vi "Teleop.vi"(10 "Match Info":T1={"Autonomous Elapsed Seconds"=0.0, "TeleOp Elapsed Seconds"=0.0, "Disabled Elapsed Seconds"=0.0, "Visited Autonomous"=FALSE, "Visited TeleOp"=FALSE, "Visited Disabled"=FALSE, "Autonomous Settings"={"Autonomous Style"=enum."Independent", "VI Refnum"=refnum}}, 11 "Call Context":T2) -> ()   [LabVIEW 2017]
doc: "This VI is called for each TeleOp packet received from the DS where the robot is not disabled. It is often used to read from the joysticks and update I/O or to update setpoints for timed control loops. It should complete and return within 20 milliseconds or it may miss DS packets."
uses:
  <vilib>/Rock Robotics/WPI/DriverStation/WPI_DriverStationDerivedRobotMode.ctl
  <vilib>/Rock Robotics/WPI/DriverStation/WPI_DriverStationMatch Info.ctl
  <vilib>/Rock Robotics/WPI/Utilities/WPI_GetSetVariantRefNum.vi
  <vilib>/Rock Robotics/Network Tables/NT Write Boolean Array.vi
  <vilib>/Rock Robotics/Network Tables/NT Write Numeric Array.vi
  <vilib>/Rock Robotics/Network Tables/NT Read Boolean.vi
  <vilib>/Rock Robotics/Network Tables/NT Read Number.vi
panel:
  out "Sample Boolean 3":bool
  out "Sample Boolean 2":bool
  out "Sample Slider 1":dbl(slide) scale=0.0..5.0
  out "Left axis value":dbl
  out "Right axis value":dbl
  in  "Square Inputs":bool
  out "Left Motor Value":dbl
  out "Right Motor Value":dbl
  in  "Max Output":dbl
  out "Sample Slider 0":dbl(slide) scale=0.0..5.0
  out "Sample Boolean 1":bool
  out "Sample Boolean 0":bool
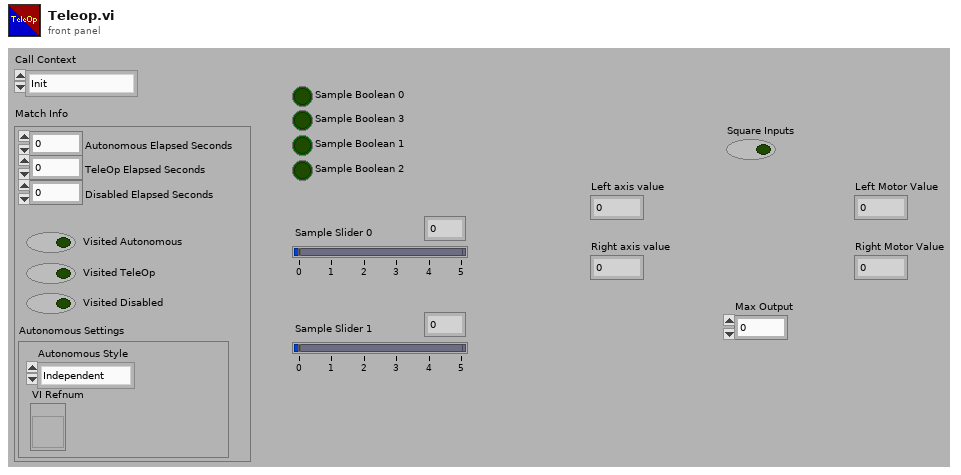
[diagram p1: front panel]
types:
  T1 = typedef "WPI_DriverStationMatch Info.ctl" = cluster{"Autonomous Elapsed Seconds":dbl, "TeleOp Elapsed Seconds":dbl, "Disabled Elapsed Seconds":dbl, "Visited Autonomous":bool, "Visited TeleOp":bool, "Visited Disabled":bool, "Autonomous Settings":cluster{"Autonomous Style":enum16{"Iterative", "Independent"}, "VI Refnum":refnum<vi>}}
  T2 = typedef "WPI_DriverStationDerivedRobotMode.ctl" = enum16{"Init", "Execute", "Stop"}
  T3 = typedef "WPI_JoystickDevRef.ctl" = cluster{"Device":T4}
  T4 = typedef "WPI_JoystickDeviceEnum.ctl" = enum16{"USB 0", "USB 1", "USB 2", "USB 3", "USB 4", "USB 5"}
  T5 = typedef "WPI_MotorControlDeviceRef.ctl" = cluster{"DeviceStatus":errorcluster, "Type":T6, "PWM":cluster{"PWM Channel":T7, "DeadBand":T8}, "CAN":cluster{"Device Number":u8, "SetOutput VI Ref":variant, "GetOutput VI Ref":variant, "Enable VI Ref":variant, "Disable VI Ref":variant, "Data":variant}, "Invert":bool, "DIO PWM":cluster{"PWM \"Enable\" Channel":T7, "DIOChannel":T9, "PWM Rate":dbl}}
  T6 = typedef "WPI_MotorControlType.ctl" = enum16{"PWM", "CAN", "DIO PWM"}
  T7 = typedef "FPGA_DIOPWMChannel.ctl" = enum8{"PWM 0", "PWM 1", "PWM 2", "PWM 3", "PWM 4", "PWM 5", "PWM 6", "PWM 7", "PWM 8", "PWM 9", "PWM MXP 0", "PWM MXP 1", "PWM MXP 2", "PWM MXP 3", "PWM MXP 4", "PWM MXP 5", "PWM MXP 6", "PWM MXP 7", "PWM MXP 8", "PWM MXP 9", "Invalid"}
  T8 = typedef "WPI_PWMDeadband.ctl" = cluster{"Name":string, "maxPositivePwm":i32, "minPositivePwm":i32, "centerPwm":i32, "maxNegativePwm":i32, "minNegativePwm":i32, "angularRange":u16}
  T9 = typedef "FPGA_DIOChannel.ctl" = enum8{"DIO 0", "DIO 1", "DIO 2", "DIO 3", "DIO 4", "DIO 5", "DIO 6", "DIO 7", "DIO 8", "DIO 9", "DIO MXP 0", "DIO MXP 1", "DIO MXP 2", "DIO MXP 3", "DIO MXP 4", "DIO MXP 5", "DIO MXP 6", "DIO MXP 7", "DIO MXP 8", "DIO MXP 9", "DIO MXP 10", "DIO MXP 11", "DIO MXP 12", "DIO MXP 13", "DIO MXP 14", "DIO MXP 15", "SPI Port CS1", "SPI Port CS2", "SPI Port CS3", "SPI Port MISO", "SPI Port MOSI", "Invalid"}
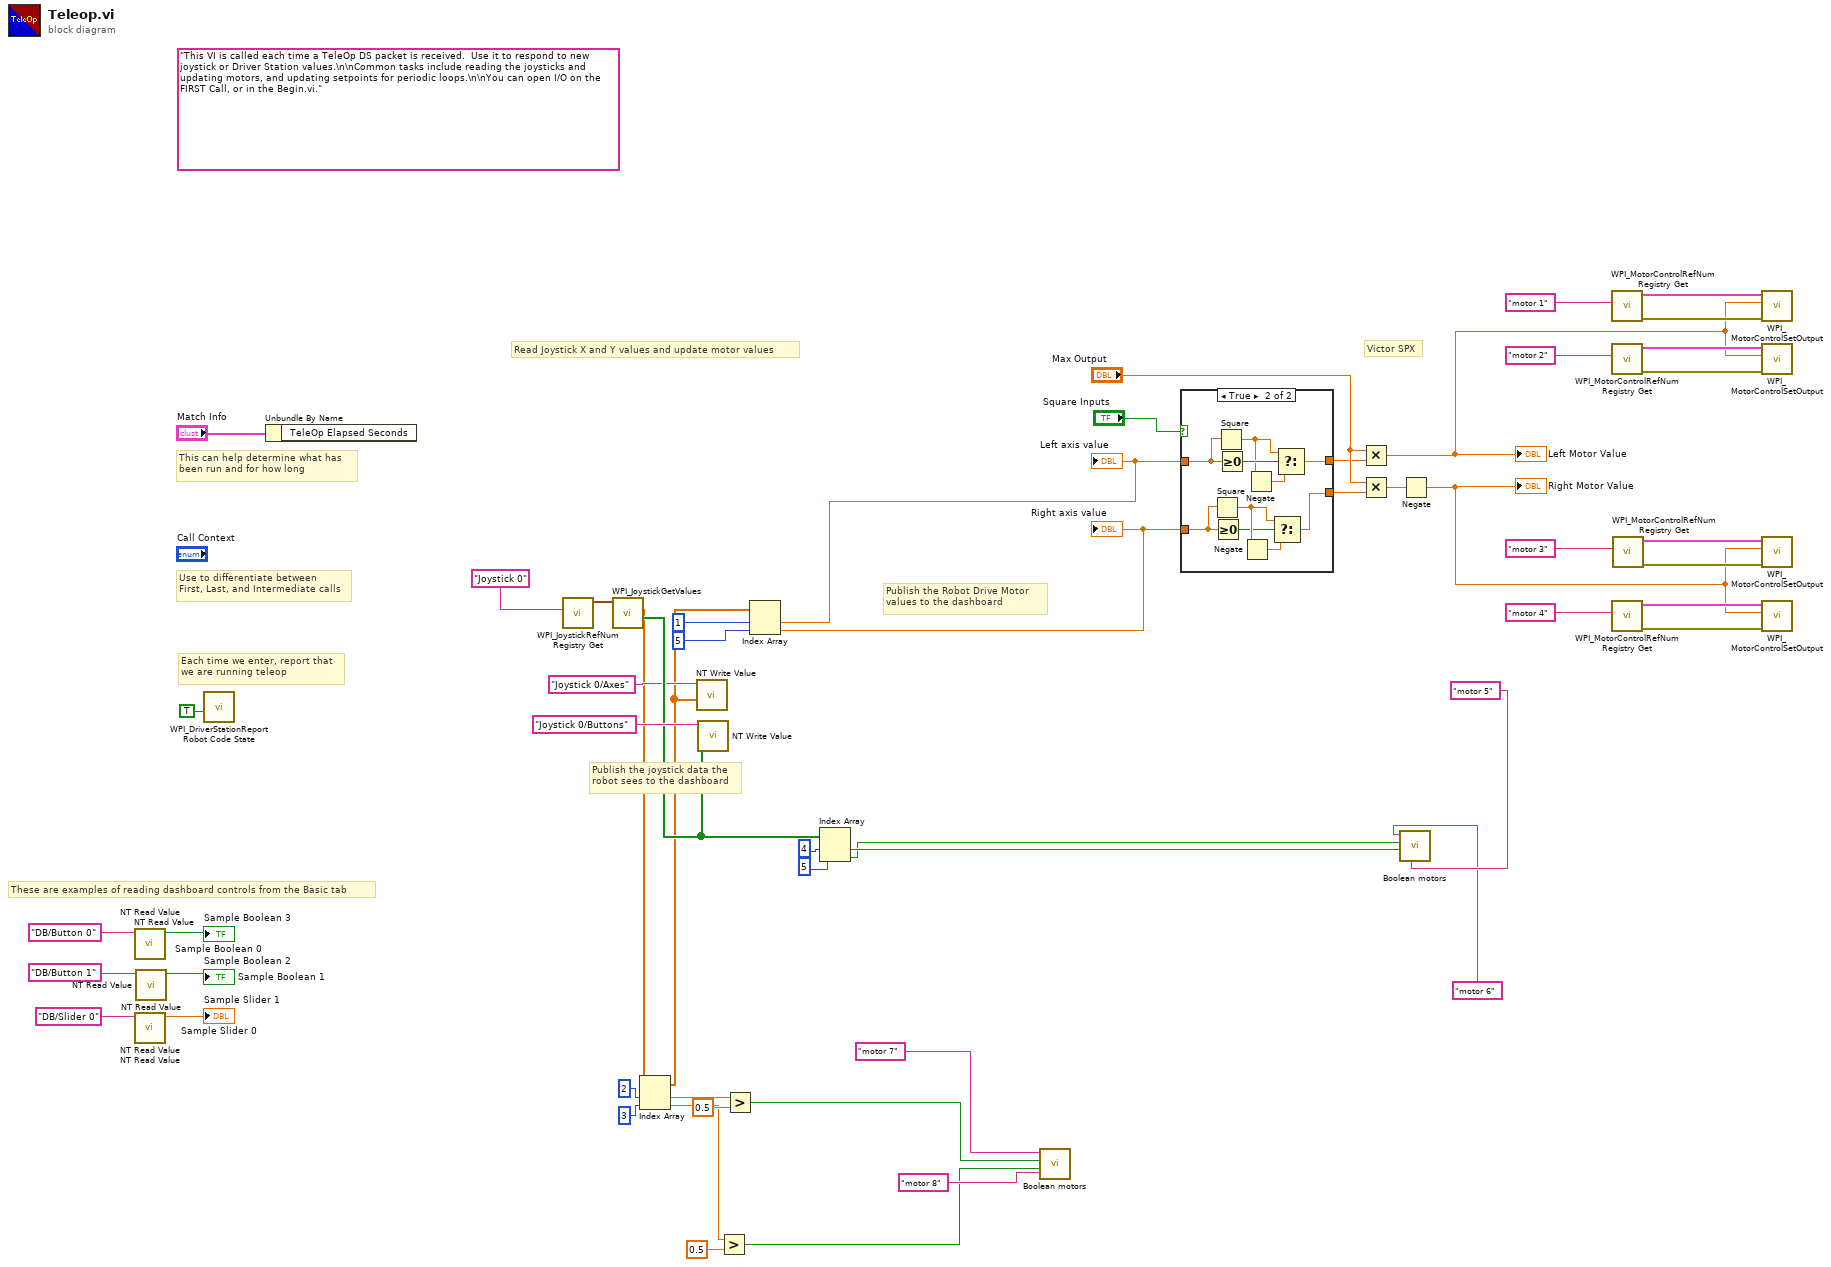
[diagram p0: block diagram]
diagram:
  (unwired) "This VI is called each time a TeleOp DS packet is received.  Use it to respond to new joystick or Driver Station values.\n\nCommon tasks include reading the joysticks and updating motors, and updating setpoints for periodic loops.\n\nYou can open I/O on the FIRST Call, or in the Begin.vi."
  # "These are examples of reading dashboard controls from the Basic tab"
  # "Victor SPX"
  # "These are examples of reading dashboard controls from the Basic tab"
  # "Publish the Robot Drive Motor\nvalues to the dashboard"
  # "Publish the joystick data the\nrobot sees to the dashboard"
  # "Each time we enter, report that\nwe are running teleop"
  # "Use to differentiate between\nFirst, Last, and Intermediate calls"
  # "This can help determine what has\nbeen run and for how long"
  # "Read Joystick X and Y values and update motor values"
  n1 = call-poly <vilib>:"NT Read Value.vi"("Name"="DB/Button 0" ("refnum name")) -> ("Boolean"=→"Sample Boolean 3":bool)  [unwired: 9 in, 1 out]
  n2 = call-poly <vilib>:"NT Read Value.vi"("Name"="DB/Button 0" ("refnum name")) -> ("Boolean"=→"Sample Boolean 0":bool)  [unwired: 9 in, 1 out]
  n3 = call-poly <vilib>:"NT Read Value.vi"("Name"="DB/Slider 0" ("refnum name")) -> ("Numeric"=→"Sample Slider 1":dbl)  [unwired: 9 in, 1 out]
  n4 = call-poly <vilib>:"NT Read Value.vi"("Name"="DB/Slider 0" ("refnum name")) -> ("Numeric"=→"Sample Slider 0":dbl)  [unwired: 9 in, 1 out]
  n5 = call-poly <vilib>:"NT Read Value.vi"("Name"="DB/Button 1" ("refnum name")) -> ("Boolean"=→"Sample Boolean 2":bool)  [unwired: 9 in, 1 out]
  n6 = call-poly <vilib>:"NT Read Value.vi"("Name"="DB/Button 1" ("refnum name")) -> ("Boolean"=→"Sample Boolean 1":bool)  [unwired: 9 in, 1 out]
  n7 = call <vilib>:"WPI_DriverStationReport Robot Code State.vi"("TeleOp"=TRUE ("Autonomous")) -> ()  [unwired: 10 in, 1 out]
  n8 = Unbundle By Name("Match Info") -> ()  [unwired: 1 out]
  n9 = call <vilib>:"WPI_JoystickRefNum Registry Get.vi"("refnum name"="Joystick 0") -> ("JoystickDevRef"=w57:T3)  [unwired: 1 in, 9 out]
  n10 = call <vilib>:"WPI_JoystickGetValues.vi"("JoystickDevRef"=w57) -> ("Buttons"=w21:bool[], "Axes"=w9:dbl[])  [unwired: 6 in, 3 out]
  n11 = Index Array(array=w9, index #1=2 ("index"), index #2=3 ("index")) -> (element #1=w8:dbl, element #2=w6:dbl)
  n12 = call-poly <vilib>:"NT Write Value.vi"("Numeric Array"=w9, "Name"="Joystick 0/Axes") -> ()  [unwired: 9 in, 1 out]
  n13 = call-poly <vilib>:"NT Write Value.vi"("Boolean Array"=w21, "Name"="Joystick 0/Buttons") -> ()  [unwired: 9 in, 1 out]
  n14 = Greater?(x=w6, y=0.5) -> (0:w1:bool)
  n15 = Greater?(x=w8, y=0.5) -> (0:w2:bool)
  n16 = Index Array(array=w9, index #1=1 ("index"), index #2=5 ("index")) -> (element #1=w39:dbl, element #2=w38:dbl)
  "Right axis value" <- w38
  "Left axis value" <- w39
  n17 = Index Array(array=w21, index #1=4 ("index"), index #2=5 ("index")) -> (element #1=w20:bool, element #2=w19:bool)
  n18 = call "Boolean motors.vi"("right motor"="motor 8" ("refnum name"), "right input"=w1, "left input"=w2, "left motor"="motor 7" ("refnum name")) -> ()  [unwired: 8 in]
  n19 = case shown="True" "Square Inputs" {
    tunnel: w39 -> [w61 w71]
    tunnel: [w61 w67] -> w42
    tunnel: [w60 w63] -> w44
    tunnel: w38 -> [w60 w62]
    frame False {
    }
    frame True {
      n20 = Square(x=w62) -> (x^2=w65:dbl)
      n21 = Greater Or Equal To 0?(x=w62) -> (x >= 0?=w64:bool)
      n22 = Square(x=w71) -> (x^2=w69:dbl)
      n23 = Greater Or Equal To 0?(x=w71) -> (x >= 0?=w70:bool)
      n24 = Negate(x=w65) -> (-x=w66:dbl)
      n25 = Negate(x=w69) -> (-x=w68:dbl)
      n26 = Select(t=w65, s=w64, f=w66) -> (s? t:f=w63:dbl)
      n27 = Select(t=w69, s=w70, f=w68) -> (s? t:f=w67:dbl)
    }
  }
  n28 = Multiply(x="Max Output", y=w42) -> (x*y=w28:dbl)
  "Left Motor Value" <- w28
  n29 = Multiply(x="Max Output", y=w44) -> (x*y=w26:dbl)
  n30 = call "Boolean motors.vi"("right motor"="motor 5" ("refnum name"), "right input"=w20, "left input"=w19, "left motor"="motor 6" ("refnum name")) -> ()  [unwired: 8 in]
  n31 = Negate(x=w26) -> (-x=w27:dbl)
  "Right Motor Value" <- w27
  n32 = call <vilib>:"WPI_MotorControlRefNum Registry Get.vi"("refnum name"="motor 1") -> ("error out"=w47:errorcluster, "MotorControlDevRef"=w46:T5)  [unwired: 9 in]
  n33 = call <vilib>:"WPI_MotorControlRefNum Registry Get.vi"("refnum name"="motor 2") -> ("error out"=w36:errorcluster, "MotorControlDevRef"=w37:T5)  [unwired: 9 in]
  n34 = call <vilib>:"WPI_MotorControlRefNum Registry Get.vi"("refnum name"="motor 4") -> ("error out"=w30:errorcluster, "MotorControlDevRef"=w31:T5)  [unwired: 9 in]
  n35 = call <vilib>:"WPI_MotorControlRefNum Registry Get.vi"("refnum name"="motor 3") -> ("error out"=w33:errorcluster, "MotorControlDevRef"=w32:T5)  [unwired: 9 in]
  n36 = call <vilib>:"WPI_MotorControlSetOutput.vi"("error in (no error)"=w47, "Output"=w28, "MotorControlDevRef"=w46) -> ()  [unwired: 6 in, 3 out]
  n37 = call <vilib>:"WPI_MotorControlSetOutput.vi"("error in (no error)"=w36, "Output"=w28, "MotorControlDevRef"=w37) -> ()  [unwired: 6 in, 3 out]
  n38 = call <vilib>:"WPI_MotorControlSetOutput.vi"("error in (no error)"=w33, "Output"=w27, "MotorControlDevRef"=w32) -> ()  [unwired: 6 in, 3 out]
  n39 = call <vilib>:"WPI_MotorControlSetOutput.vi"("error in (no error)"=w30, "Output"=w27, "MotorControlDevRef"=w31) -> ()  [unwired: 6 in, 3 out]
